vi "留样信息存储.vi"() -> ()   [LabVIEW 2016, in "德润DR803L超标留样.lvlib"]
uses:
  <vilib>/addons/database/Auxilliary.llb/DB Tools Column Info.ctl
  <vilib>/addons/database/Auxilliary.llb/DB Tools DataTypes.ctl
  <vilib>/addons/database/NI_Database_API.lvlib
  <vilib>/Utility/VariantDataType/VariantType.lvlib
panel:
  out "data输出":T1
  out "数组":string[](array[string])
  out "电子表格字符串":string
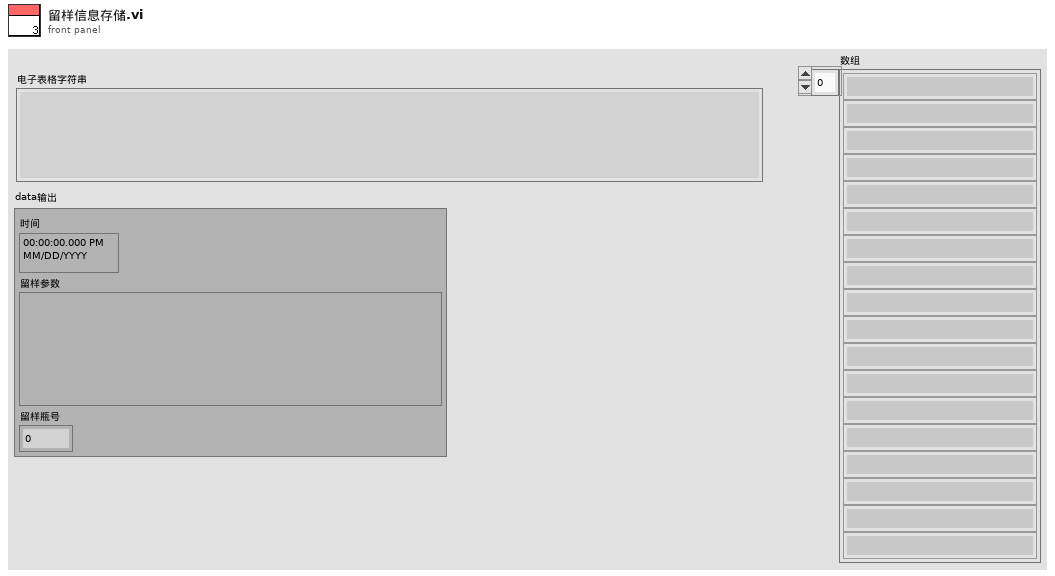
[diagram p1: front panel]
types:
  T1 = cluster{"时间":timestamp, "留样参数":string, "留样瓶号":dbl}
  T2 = enum16{"open", "read", "write", "write single", "close"}
  T3 = typedef "NI_Database_API.lvlib/DB Tools Column Info.ctl" = cluster{"column name":string, "data type":T4, "size":i32, "allow null?":bool}
  T4 = typedef "NI_Database_API.lvlib/DB Tools DataTypes.ctl" = enum16{"String", "Long (I32)", "Single (SGL)", "Double (DBL)", "Date/Time", "Binary"}
  T5 = cluster{"采样器状态":enum16{"停止", "运行"}, "当前留样瓶编号":u16, "报警状态":enum16{"无报警", "缺水报警"}, "超标信号":enum16{"无信号", "超标信号"}, "采样器进程":enum16{"停止", "待机", "定位校正", "移除瓶盖", "采样瓶排空", "管路润洗", "管存", "进样", "瓶盖密封", "管路排空", "调整采样位置", "采样结束", "采样瓶润洗", "瓶润洗排空"}, "版本号":string, "同步信号":enum16{"无信号", "同步信号"}, "外控信号":enum16{"无信号", "外控信号"}, "门状态":enum16{"门开", "门关"}, "当前瓶号":u16, "工作状态":enum16{"停止", "采样中"}, "留样模式":enum16{"无", "定时留样", "时间等比例", "超标留样", "同步留样", "外控留样"}, "立即留样":enum16{"无", "远程留样"}, "采样方式":enum16{"单采", "双重"}, "仪器时间":timestamp, "单次采样量":u16, "时间等比采样采样间隔":u16, "排空命令":u16, "远程复位":u16, "门禁密码":u16}
  T6 = typedef "VariantType.lvlib/Type.ctl" = enum8{"Invalid Type", "Void", "I8", "I16", "I32", "I64", "U8", "U16", "U32", "U64", "Single Float", "Double Float", "Extended Float", "Single Complex", "Double Complex", "Extended Complex", "Enum U8", "Enum U16", "Enum U32", "Enum U64", "Single Float With Unit", "Double Float With Unit", "Extended Float With Unit", "Single Complex with Unit", "Double Complex with Unit", "Extended Complex with Unit", "Boolean", "String", "Path", "Picture", "Tag", "Array", "Cluster", "Variant", "LV Variant", "Waveform", "Timestamp", "Digital Waveform", "Digital Data", "ExpressData", "Refnum", "External Data", "VI", "Poly VI", "LabVIEW Class Instance", "Fixed Point"}
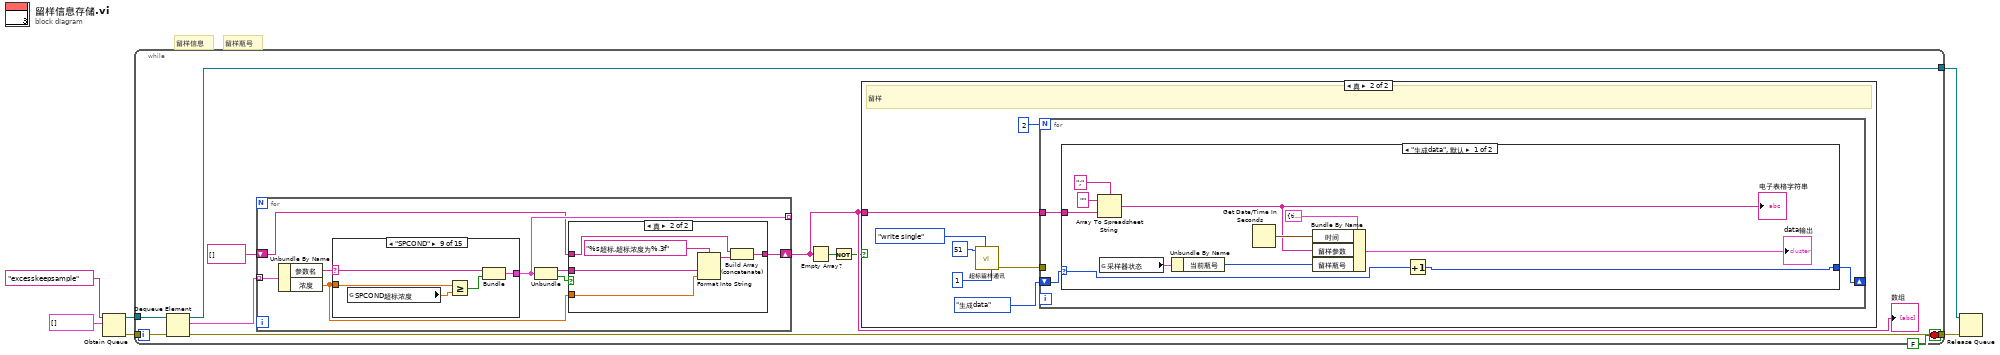
[diagram p0: block diagram]
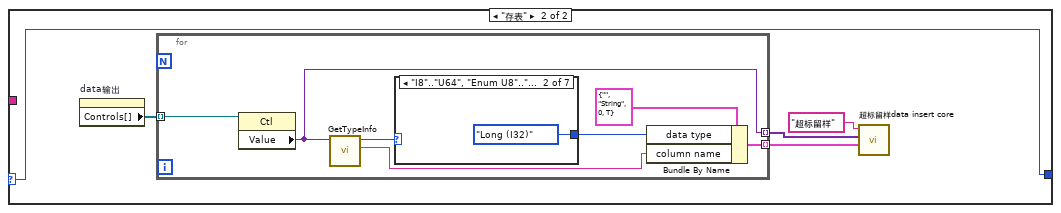
[diagram p3: hidden frame]
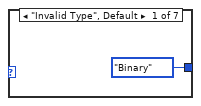
[diagram p4: hidden frame]
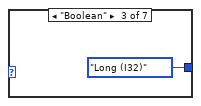
[diagram p5: hidden frame]
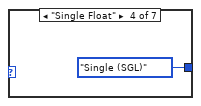
[diagram p6: hidden frame]
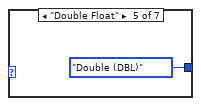
[diagram p7: hidden frame]
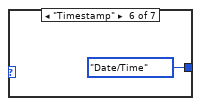
[diagram p8: hidden frame]
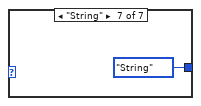
[diagram p9: hidden frame]
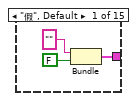
[diagram p11: hidden frame]
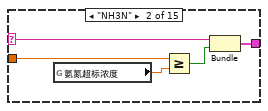
[diagram p12: hidden frame]
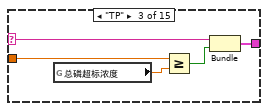
[diagram p13: hidden frame]
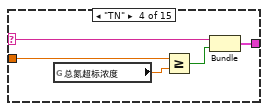
[diagram p14: hidden frame]
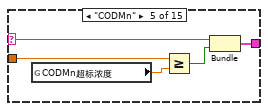
[diagram p15: hidden frame]
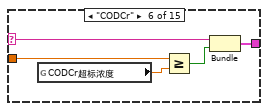
[diagram p16: hidden frame]
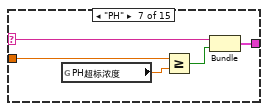
[diagram p17: hidden frame]
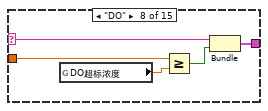
[diagram p18: hidden frame]
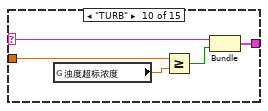
[diagram p19: hidden frame]
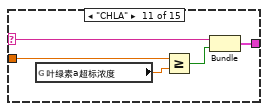
[diagram p20: hidden frame]
diagram:
  # "留样信息"
  # "留样瓶号"
  n1 = Obtain Queue(name (unnamed)="excesskeepsample" ("名称（未命名）"), element data type=cluster{"参数名":string, "浓度":dbl}[] []) -> (queue out=w4:refnum<queue>, error out=w3:errorcluster)  [unwired: 3 in, 1 out]
  n2 = while {
    tunnel: w4 -> [w16]
    tunnel: w3 -> [w14]
    tunnel: [w13] -> w2
    tunnel: [w12] -> w1
    stop <- FALSE stop-if-true
    n3 = Dequeue Element(queue=w16, error in (no error)=w14) -> (queue out=w13:refnum<queue>, element=w11:cluster{"参数名":string, "浓度":dbl}[], error out=w12:errorcluster)  [unwired: 1 in, 1 out]
    n4 = for {
      tunnel: w11 -> [w64] mode=indexing
      tunnel: [w61] -> _ mode=indexing
      shift-right: [w58] -> w9
      shift-left: string[] [] -> [w57]
      n5 = Unbundle By Name(w64) -> ("参数名"=w63:string, "浓度"=w62:dbl)
      n6 = case shown="\"SPCOND\"" w63 {
        selector: w63 -> [_ w77 w81 w86 w92 w97 w102 w107 w112 w117 w122 w127 w132 w137 w141]
        tunnel: w62 -> [_ w79 w82 w87 w93 w98 w103 w108 w113 w118 w123 w128 w133 w138 w140]
        tunnel: [w72 w75 w80 w85 w91 w96 w101 w106 w111 w116 w121 w126 w131 w136 w143] -> w61
        frame "假", Default {
          n7 = Bundle("", FALSE) -> (w72:cluster{string, bool})  [unwired: 1 in]
        }
        frame "NH3N" {
          n8 = global read "串口参数断电保存全局变量.vi" "氨氮超标浓度"() -> (w78:dbl)
          n9 = Greater Or Equal?(x=w79, y=w78) -> (x >= y?=w76:bool)
          n10 = Bundle(w77, w76) -> (w75:cluster{string, bool})  [unwired: 1 in]
        }
        frame "TP" {
          n11 = global read "串口参数断电保存全局变量.vi" "总磷超标浓度"() -> (w84:dbl)
          n12 = Greater Or Equal?(x=w82, y=w84) -> (x >= y?=w83:bool)
          n13 = Bundle(w81, w83) -> (w80:cluster{string, bool})  [unwired: 1 in]
        }
        frame "TN" {
          n14 = global read "串口参数断电保存全局变量.vi" "总氮超标浓度"() -> (w89:dbl)
          n15 = Greater Or Equal?(x=w87, y=w89) -> (x >= y?=w88:bool)
          n16 = Bundle(w86, w88) -> (w85:cluster{string, bool})  [unwired: 1 in]
        }
        frame "CODMn" {
          n17 = global read "串口参数断电保存全局变量.vi" "CODMn超标浓度"() -> (w94:dbl)
          n18 = Greater Or Equal?(x=w93, y=w94) -> (x >= y?=w90:bool)
          n19 = Bundle(w92, w90) -> (w91:cluster{string, bool})  [unwired: 1 in]
        }
        frame "CODCr" {
          n20 = global read "串口参数断电保存全局变量.vi" "CODCr超标浓度"() -> (w99:dbl)
          n21 = Greater Or Equal?(x=w98, y=w99) -> (x >= y?=w95:bool)
          n22 = Bundle(w97, w95) -> (w96:cluster{string, bool})  [unwired: 1 in]
        }
        frame "PH" {
          n23 = global read "串口参数断电保存全局变量.vi" "PH超标浓度"() -> (w104:dbl)
          n24 = Greater Or Equal?(x=w103, y=w104) -> (x >= y?=w100:bool)
          n25 = Bundle(w102, w100) -> (w101:cluster{string, bool})  [unwired: 1 in]
        }
        frame "DO" {
          n26 = global read "串口参数断电保存全局变量.vi" "DO超标浓度"() -> (w109:dbl)
          n27 = Greater Or Equal?(x=w108, y=w109) -> (x >= y?=w105:bool)
          n28 = Bundle(w107, w105) -> (w106:cluster{string, bool})  [unwired: 1 in]
        }
        frame "SPCOND" {
          n29 = global read "串口参数断电保存全局变量.vi" "SPCOND超标浓度"() -> (w114:dbl)
          n30 = Greater Or Equal?(x=w113, y=w114) -> (x >= y?=w110:bool)
          n31 = Bundle(w112, w110) -> (w111:cluster{string, bool})  [unwired: 1 in]
        }
        frame "TURB" {
          n32 = global read "串口参数断电保存全局变量.vi" "浊度超标浓度"() -> (w119:dbl)
          n33 = Greater Or Equal?(x=w118, y=w119) -> (x >= y?=w115:bool)
          n34 = Bundle(w117, w115) -> (w116:cluster{string, bool})  [unwired: 1 in]
        }
        frame "CHLA" {
          n35 = global read "串口参数断电保存全局变量.vi" "叶绿素a超标浓度"() -> (w124:dbl)
          n36 = Greater Or Equal?(x=w123, y=w124) -> (x >= y?=w120:bool)
          n37 = Bundle(w122, w120) -> (w121:cluster{string, bool})  [unwired: 1 in]
        }
        frame "ALGAL" {
          n38 = global read "串口参数断电保存全局变量.vi" "藻密度超标浓度"() -> (w129:dbl)
          n39 = Greater Or Equal?(x=w128, y=w129) -> (x >= y?=w125:bool)
          n40 = Bundle(w127, w125) -> (w126:cluster{string, bool})  [unwired: 1 in]
        }
        frame "Cyanobacteria" {
          n41 = global read "串口参数断电保存全局变量.vi" "蓝绿藻超标浓度"() -> (w134:dbl)
          n42 = Greater Or Equal?(x=w133, y=w134) -> (x >= y?=w130:bool)
          n43 = Bundle(w132, w130) -> (w131:cluster{string, bool})  [unwired: 1 in]
        }
        frame "ORP" {
          n44 = global read "串口参数断电保存全局变量.vi" "ORP超标浓度"() -> (w139:dbl)
          n45 = Greater Or Equal?(x=w138, y=w139) -> (x >= y?=w135:bool)
          n46 = Bundle(w137, w135) -> (w136:cluster{string, bool})  [unwired: 1 in]
        }
        frame "COD" {
          n47 = global read "串口参数断电保存全局变量.vi" "COD超标浓度"() -> (w144:dbl)
          n48 = Greater Or Equal?(x=w140, y=w144) -> (x >= y?=w142:bool)
          n49 = Bundle(w141, w142) -> (w143:cluster{string, bool})  [unwired: 1 in]
        }
      }
      n50 = Unbundle(w61) -> (w59:string, w60:bool)
      n51 = case shown="真" w60 {
        tunnel: w59 -> [_ w71]
        tunnel: w62 -> [_ w70]
        tunnel: [w65 w66] -> w58
        tunnel: w57 -> [w65 w68]
        frame False {
        }
        frame True {
          n52 = Format Into String(format string="%s超标,超标浓度为%.3f" ("格式字符串"), w71, w70) -> (resulting string=w67:string)  [unwired: 2 in, 1 out]
          n53 = Build Array (concatenate)(w68, w67) -> (w66:string[])
        }
      }
    }
    "数组" <- w9
    n54 = Empty Array?(array=w9) -> (empty?=w8:bool)
    n55 = Not(x=w8) -> (.not. x?=w7:bool)
    n56 = case shown="真" w7 {
      tunnel: w9 -> [_ w21]
      frame False {
      }
      frame True {
        # "留样"
        n57 = call "超标留样通讯.vi"("value"=u16 1 ("新元素/子数组"), "STEP"=T2."write single", "starting address"=51 ("索引")) -> ("error out"=w17:errorcluster)  [unwired: 6 in, 2 out]
        n58 = for {
          N: 2 -> [_]
          tunnel: w21 -> [w25]
          shift-right: [w24] -> _
          shift-left: enum16{"生成data", "存表"}."生成data" -> [w26]
          tunnel: w17 -> [_]
          n59 = case shown="\"生成data\", 默认" w26 {
            selector: w26 -> [w33 w38]
            tunnel: w25 -> [w34 _]
            tunnel: [w32 w38] -> w24
            frame "生成data", Default {
              n60 = Array To Spreadsheet String(delimiter (Tab)=";" ("分隔符(Tab)"), array=w34, 3:"") -> (spreadsheet string=w30:string)
              "电子表格字符串" <- w30
              n61 = global read "超标留样全局.vi" "采样器状态"() -> (w36:T5)
              n62 = Unbundle By Name(w36) -> ("当前瓶号"=w29:u16)
              n63 = Get Date/Time In Seconds() -> (seconds since 1Jan1904=w37:timestamp)
              n64 = Bundle By Name(cluster=T1 {"时间"=timestamp(3687928779.282504 s since 1904-01-01), "留样参数"="NH3N超标,超标浓度为0.000\r\n留样瓶号:0", "留样瓶号"=0.0} ("data输出"), "时间"=w37, "留样参数"=w30, "留样瓶号"=w29) -> (→"data输出":T1)
              n65 = Increment(x=w33) -> (x+1=w32:enum16{"生成data", "存表"})
            }
            frame "存表" {
              n66 = property on="data输出" class="Clust (严格)"() -> ("Controls[]"=w42:refnum<vi>[])  [unwired: 2 in, 2 out]
              n67 = for {
                tunnel: w42 -> [w49] mode=indexing
                tunnel: [w43] -> w40 mode=indexing
                tunnel: [w44] -> w39 mode=indexing
                n68 = property class="Ctl"(reference=w49) -> ("Value"=w43:variant)  [unwired: 1 in, 2 out]
                n69 = call <vilib>:"GetTypeInfo.vi"("Variant"=w43) -> ("Name"=w47:string, "Type Enum"=w46:T6)  [unwired: 6 in, 3 out]
                n70 = case shown="\"I8\"..\"U64\", \"Enum U8\"..\"Enum U64\"" w46 {
                  tunnel: [DB_Tools_DataTypes."Binary" ("data type") DB_Tools_DataTypes."Long (I32)" ("data type") DB_Tools_DataTypes."Long (I32)" ("data type") DB_Tools_DataTypes."Single (SGL)" ("data type") DB_Tools_DataTypes."Double (DBL)" ("data type") DB_Tools_DataTypes."Date/Time" ("data type") DB_Tools_DataTypes."String" ("data type")] -> w45
                  frame "Invalid Type", Default {
                  }
                  frame "I8".."U64", "Enum U8".."Enum U64" {
                  }
                  frame "Boolean" {
                  }
                  frame "Single Float" {
                  }
                  frame "Double Float" {
                  }
                  frame "Timestamp" {
                  }
                  frame "String" {
                  }
                }
                n71 = Bundle By Name(cluster=T3 {"column name"="", "data type"=enum."String", "size"=0, "allow null?"=TRUE} ("column information"), "data type"=w45, "column name"=w47) -> (w44:T3)
              }
              n72 = call "超标留样data insert core.vi"("column information"=w39, "data"=w40, "table"="超标留样") -> ()  [unwired: 8 in, 1 out]
            }
          }
        }
      }
    }
  }
  n73 = Release Queue(queue=w2, error in (no error)=w1) -> ()  [unwired: 1 in, 3 out]
